vi "Readable Demo.vi"() -> ()   [LabVIEW 2009]
uses:
  Lockin/Lockin SR830.lvclass
  DAQ/DAQmx Analog.lvclass
  Readable.lvclass
  Photon Counter/Photon Counter SR400.lvclass
panel:
  out "Array":dbl[](array[numeric])
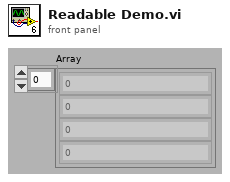
[diagram p1: front panel]
types:
  T1 = typedef "Readable.lvclass/Data Points.ctl" = T2[]
  T2 = typedef "Readable.lvclass/Data Point.ctl" = dbl
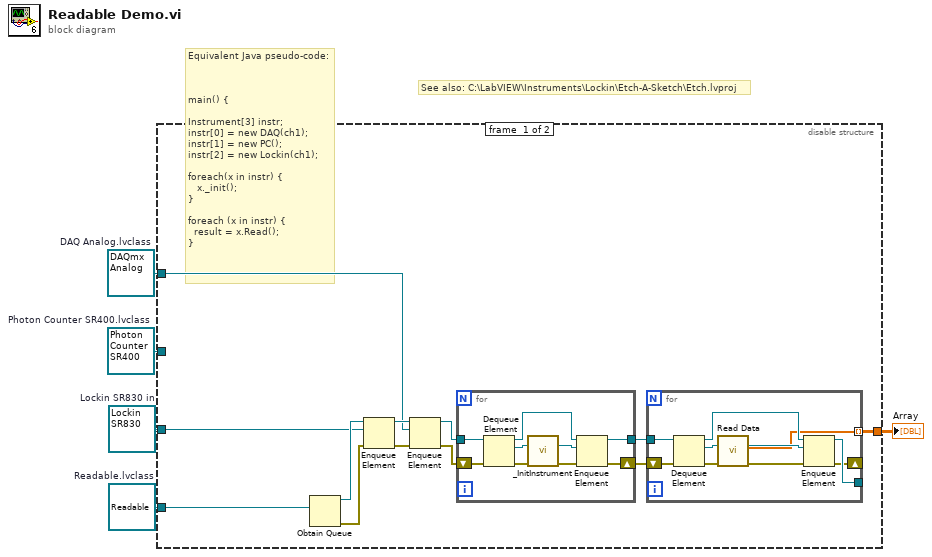
[diagram p0: block diagram]
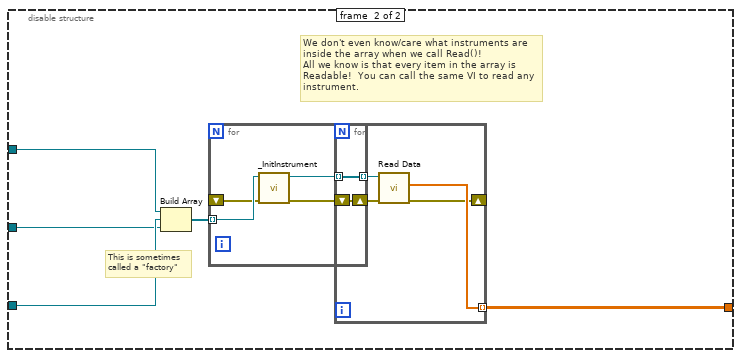
[diagram p2: hidden frame]
diagram:
  w1 = refnum<class "Photon Counter SR400.lvclass"> refnum  # Photon Counter SR400.lvclass
  w5 = refnum<class "Readable.lvclass"> refnum  # Readable.lvclass
  w3 = refnum<class "DAQmx Analog.lvclass"> refnum  # DAQ Analog.lvclass
  w4 = refnum<class "Lockin SR830.lvclass"> refnum  # Lockin SR830 in
  # "See also: C:\\LabVIEW\\Instruments\\Lockin\\Etch-A-Sketch\\Etch.lvproj"
  # "Equivalent Java pseudo-code:\n\n\n\nmain() {\n\nInstrument[3] instr;\ninstr[0] = new DAQ(ch1);\ninstr[1] = new PC();\ninstr[2] = new Lockin(ch1);\n\nforeach(x in instr) {\n   x._init();\n}\n\nforeach (x in instr) {\n  result = x.Read();\n}"
  n1 = disable-structure shown="Enabled" {
    disable-tunnel: w5 -> [w17 _]
    disable-tunnel: w4 -> [w15 w42]
    disable-tunnel: w3 -> [w13 w43]
    disable-tunnel: [w6 w39] -> w2
    disable-tunnel: w1 -> [_ w37]
    frame #0 {
      n2 = Obtain Queue(element data type=w17) -> (queue out=w16:refnum<queue>, error out=w8:errorcluster)  [unwired: 4 in, 1 out]
      n3 = Enqueue Element(queue=w16, element=w15, error in (no error)=w8) -> (queue out=w14:refnum<queue>, error out=w9:errorcluster)  [unwired: 1 in, 1 out]
      n4 = Enqueue Element(queue=w14, element=w13, error in (no error)=w9) -> (queue out=w12:refnum<queue>, error out=w10:errorcluster)  [unwired: 1 in, 1 out]
      n5 = for {
        tunnel: w12 -> [w36]
        tunnel: [w32] -> w11
        shift-right: [w28] -> w7
        shift-left: w10 -> [w29]
        n6 = Dequeue Element(queue=w36, error in (no error)=w29) -> (queue out=w34:refnum<queue>, element=w35:refnum<class "Readable.lvclass">, error out=w30:errorcluster)  [unwired: 1 in, 1 out]
        n7 = call-dynamic "_InitInstrument.vi"("error in (no error)"=w30, "Instrument in"=w35) -> ("error out"=w31:errorcluster, "Instrument out"=w33:refnum<class "Readable.lvclass">)  [unwired: 8 in]
        n8 = Enqueue Element(queue=w34, element=w33, error in (no error)=w31) -> (queue out=w32:refnum<queue>, error out=w28:errorcluster)  [unwired: 1 in, 1 out]
      }
      n9 = for {
        tunnel: w11 -> [w27]
        tunnel: [w25] -> _
        shift-right: [w19] -> _
        shift-left: w7 -> [w20]
        tunnel: [w18] -> w6 mode=indexing
        n10 = Dequeue Element(queue=w27, error in (no error)=w20) -> (queue out=w26:refnum<queue>, element=w24:refnum<class "Readable.lvclass">, error out=w22:errorcluster)  [unwired: 1 in, 1 out]
        n11 = call "Read Data.vi"("error in (no error)"=w22, "Readable in"=w24) -> ("error out"=w21:errorcluster, "Data Points"=w18:T1, "Readable out"=w23:refnum<class "Readable.lvclass">)  [unwired: 3 in, 4 out]
        n12 = Enqueue Element(queue=w26, element=w23, error in (no error)=w21) -> (queue out=w25:refnum<queue>, error out=w19:errorcluster)  [unwired: 1 in, 1 out]
      }
    }
    frame #1 {
      # "We don't even know/care what instruments are inside the array when we call Read()!\nAll we know is that every item in the array is  Readable!  You can call the same VI to read any instrument."
      # "This is sometimes\ncalled a \"factory\""
      n13 = Build Array(w43, w42, w37) -> (w40:refnum<class "Readable.lvclass">[])
      n14 = for {
        tunnel: [w51] -> w41 mode=indexing
        tunnel: w40 -> [w50] mode=indexing
        shift-right: [w49] -> w38
        shift-left: _ -> [w48]
        n15 = call-dynamic "_InitInstrument.vi"("error in (no error)"=w48, "Instrument in"=w50) -> ("error out"=w49:errorcluster, "Instrument out"=w51:refnum<class "Readable.lvclass">)  [unwired: 4 in, 4 out]
      }
      n16 = for {
        tunnel: w41 -> [w47] mode=indexing
        tunnel: [w46] -> w39 mode=indexing
        shift-right: [w44] -> _
        shift-left: w38 -> [w45]
        n17 = call "Read Data.vi"("error in (no error)"=w45, "Readable in"=w47) -> ("error out"=w44:errorcluster, "Data Points"=w46:T1)  [unwired: 8 out]
      }
    }
  }
  "Array" <- w2
